vi "Search for tag.vi"(0 "Directory":T1[](array[typedef]), 1 "Tag":u16) -> (2 "Tag found":T1, 3 "Byte stream offset\nwhere tag should be":i32, 4 "Tag exists?":bool)   [LabVIEW 2015, in "Tiff reader.lvlib"]
doc: "Search for a tag by Tag # in the IFD (the directory) and returns the tag and the place in the byte stream where the tag should be located."
uses:
  Tiff reader.lvlib
  FieldTypes.ctl
  IFD Entry.ctl
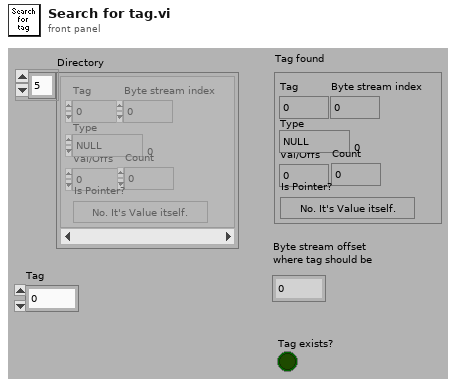
[diagram p1: front panel]
types:
  T1 = typedef "Tiff reader.lvlib/IFD Entry.ctl" = cluster{"Tag":u16, "Type":T2, "Count":u32, "Val/Offs":u32, "Is Pointer?":bool, "Byte stream index":i32}
  T2 = typedef "Tiff reader.lvlib/FieldTypes.ctl" = enum16{"NULL", "U8", "ASCII7", "U16", "U32", "RATIONAL", "SByte(I8)", "Undef(8Bit)", "I16", "I32", "SRat(4B:4B)", "SGL(4Byte)", "DBL(8Byte)"}
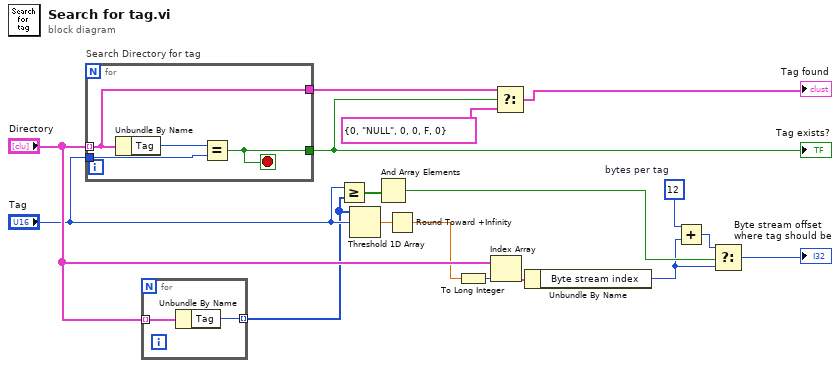
[diagram p0: block diagram]
diagram:
  w3 = 12  # bytes per tag
  n1 = for "Search Directory for tag" {
    tunnel: "Directory" -> [w19] mode=indexing
    tunnel: "Tag" -> [w21]
    tunnel: [w20] -> w17
    tunnel: [w19] -> w15
    stop <- w20 stop-if-true
    n2 = Unbundle By Name(w19) -> ("Tag"=w18:u16)
    n3 = Equal?(x=w18, y=w21) -> (x = y?=w20:bool)
  }
  "Tag exists?" <- w17
  n4 = for {
    tunnel: "Directory" -> [w23] mode=indexing
    tunnel: [w22] -> w7 mode=indexing
    n5 = Unbundle By Name(w23) -> ("Tag"=w22:u16)
  }
  n6 = Greater Or Equal?(x="Tag", y=w7) -> (x >= y?=w8:bool[])
  n7 = Threshold 1D Array(2:"Tag", 3:w7) -> (0:w13:dbl)  [unwired: 1 out]
  n8 = And Array Elements(Boolean array=w8) -> (logical AND=w4:bool)
  n9 = Round Toward +Infinity(x=w13) -> (ceil(x): smallest int >= x=w6:dbl)
  n10 = To Long Integer(number=w6) -> (32bit integer=w12:i32)
  n11 = Index Array(array="Directory", index=w12) -> (element=w11:T1)
  n12 = Select(t=w15, s=w17, f=T1 {"Tag"=0, "Type"=enum."NULL", "Count"=0, "Val/Offs"=0, "Is Pointer?"=FALSE, "Byte stream index"=0}) -> (s? t:f=→"Tag found":T1)
  n13 = Unbundle By Name(w11) -> ("Byte stream index"=w1:i32)
  n14 = Add(x=w3, y=w1) -> (x+y=w2:i32)
  n15 = Select(t=w2, s=w4, f=w1) -> (s? t:f=→"Byte stream offset\nwhere tag should be":i32)
